vi "Demo Main -translationstage.vi"() -> ()   [LabVIEW 2021]
uses:
  Logo.ctl
  <vilib>/Utility/file.llb/Write Delimited Spreadsheet (string).vi
  <vilib>/Utility/file.llb/Write Delimited Spreadsheet (I64).vi
  <vilib>/Utility/file.llb/Write Delimited Spreadsheet (DBL).vi
  <vilib>/Analysis/NI_AALBase.lvlib
panel:
  in  ".NET Container":refnum<k24>(container)
  in  "MG17Motor":refnum<k7>(container)
  out "ESD":i32=1 caption="Steps\nAdded/Removed"
  in  "ES":i32=1 caption="Add /Remove \nSteps"
  out "Sweep Graph":u32[](graph)
  out "SM":i32 caption="Sweep\nMean"
  out "SN":i32=31 caption="Current Sweep Iteration"
  out "SND":i32=31 caption="Total No. of Sweeps"
  in  "Auto-Sweep":bool
  in  "P8":bool
  out "PC":i32=186 caption="Current \nPosition"
  out "WTD":i32=10000 caption="Wait Time (ms)\nRead Data"
  out "EPD":i32=180 caption="End Position\nRead Data"
  out "SPD":i32 caption="Start Position\nRead Data"
  out "SSD":i32=6 caption="Step Size\nRead Data"
  in  "SP":i32 caption="Start Position (degrees)\n Set Data"
  in  "WT":i32=10000 caption="Wait Time (ms)\n Set Data"
  in  "EP":i32=90 caption="End Position (degrees)\n Set Data"
  in  "P7":bool
  in  "SS":dbl=3.0 caption="Step Size (degrees)\nSet Data"
  in  "Motor Controller\nSerialNumber":string="40837323"
  in  "Export":bool
  out "DB":u32[](array[numeric])=[12, 0, 0, 0, 0, 0, 0, 0, 0, 0, 0, 0, 0, 0, 0, 0]
  out "OVL":bool caption="LED ON : Over Rang Data"
  out "OLD":i32
  out "GN":i32 caption="Gate Number"
  in  "Correction":bool
  in  "Logo":T1
  out "Graph":u32[](graph)=[22]
  in  "Stop":bool
  in  "Start":bool
  in  "P6":bool
  out "RND":i32=10 caption="Read Number\nRead Data"
  in  "P5":bool
  in  "RN":i32=10 caption="Read Number\nSet Data"
  out "PowerD":i32 caption="Power\nRead Data"
  out "ITD":i32=100 caption="Internal Time\nRead Data"
  in  "P4":bool
  in  "P3":bool
  in  "IT":i32=40 caption="Internal Time\nSet Data"
  in  "P2":bool
  out "Handle Number":i32=1331832464
  in  "P1":bool caption="Switch\nPower OFF/Power ON"
  in  "EXIT":bool=TRUE
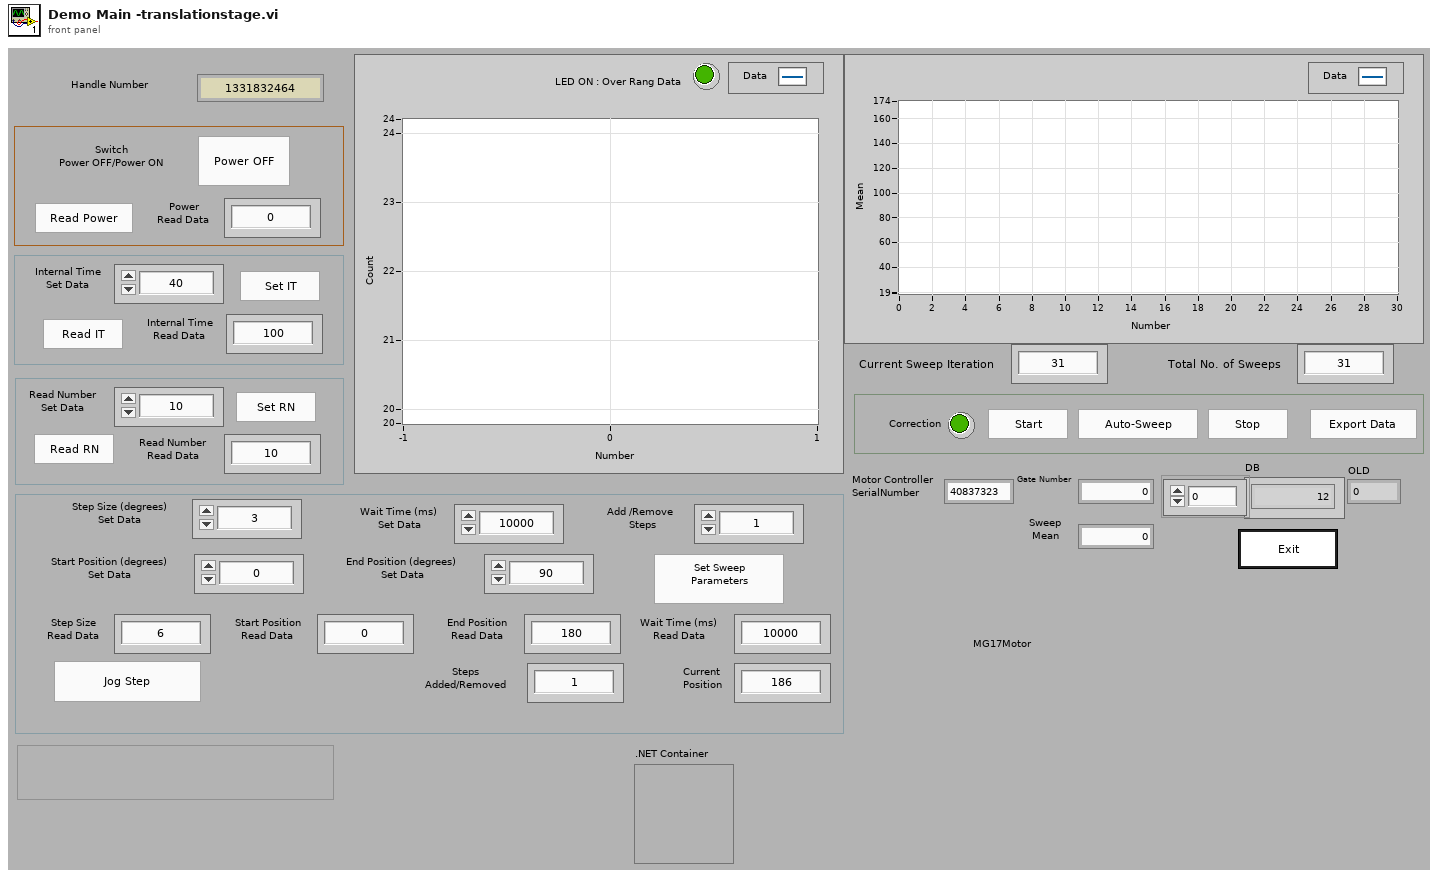
[diagram p1: front panel]
types:
  T1 = typedef "Logo.ctl" = bool
  T2 = enum8{"Enabled", "Disabled", "Disabled and Grayed Out"}
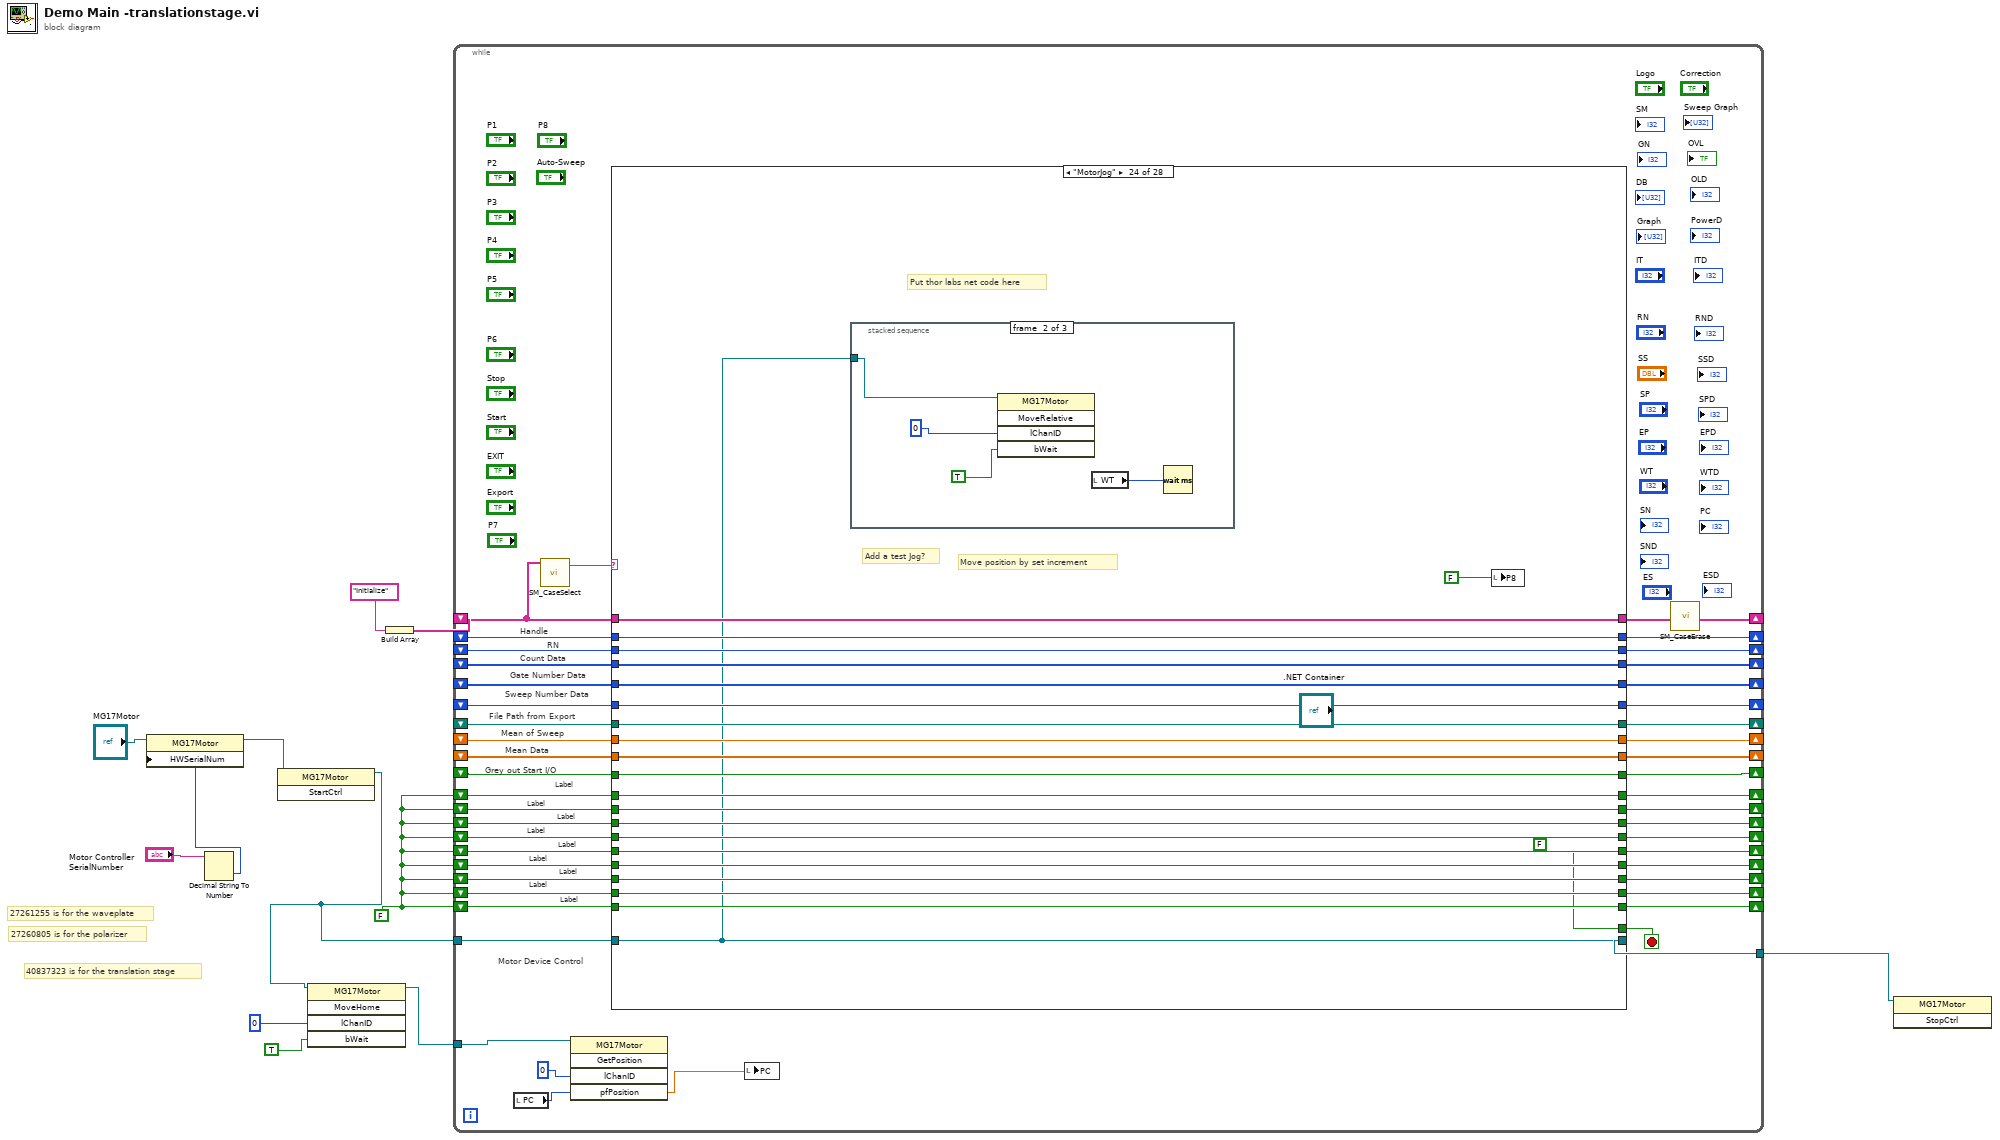
[diagram p0: block diagram]
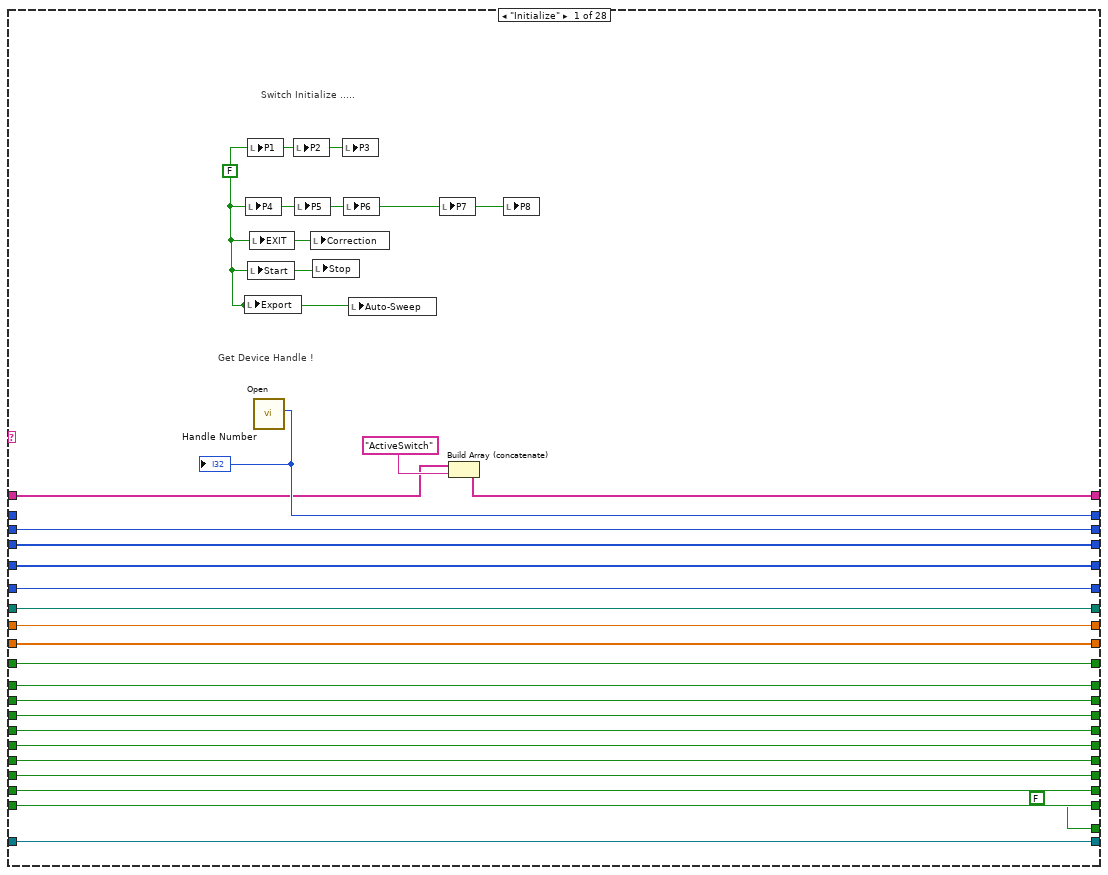
[diagram p2: hidden frame]
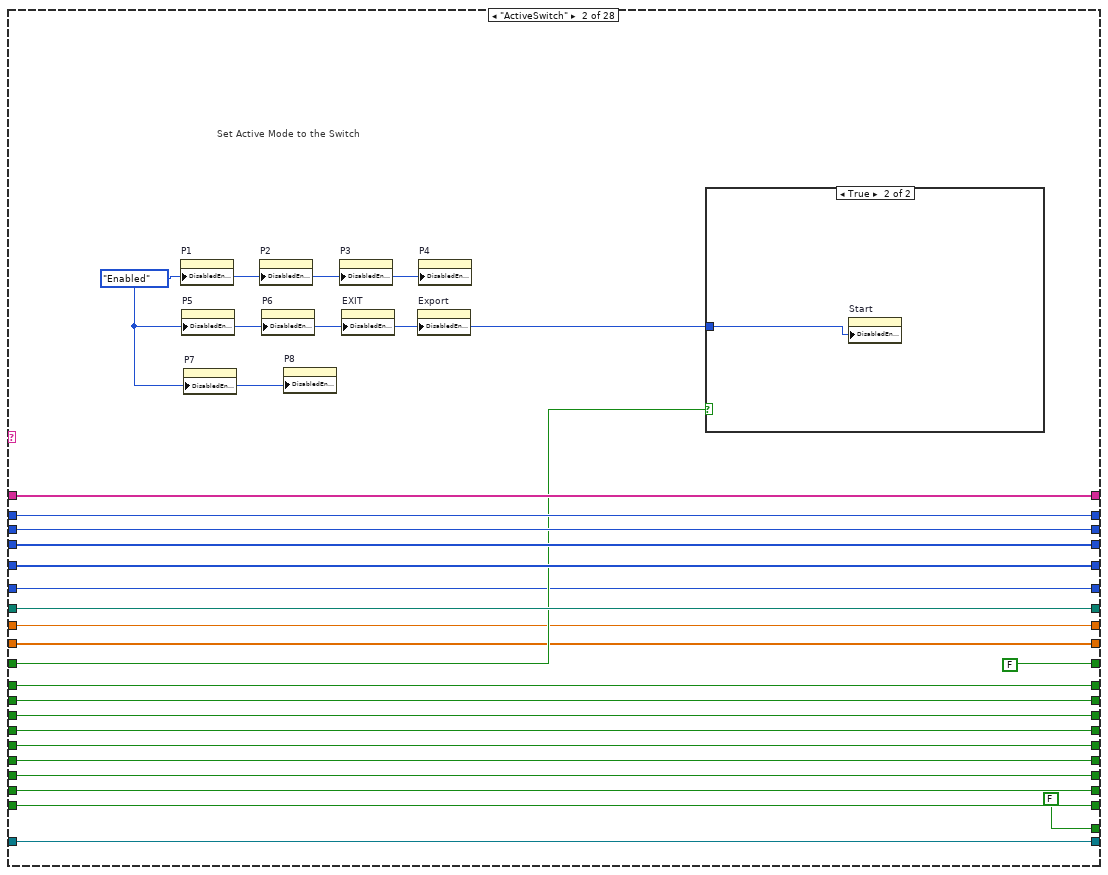
[diagram p3: hidden frame]
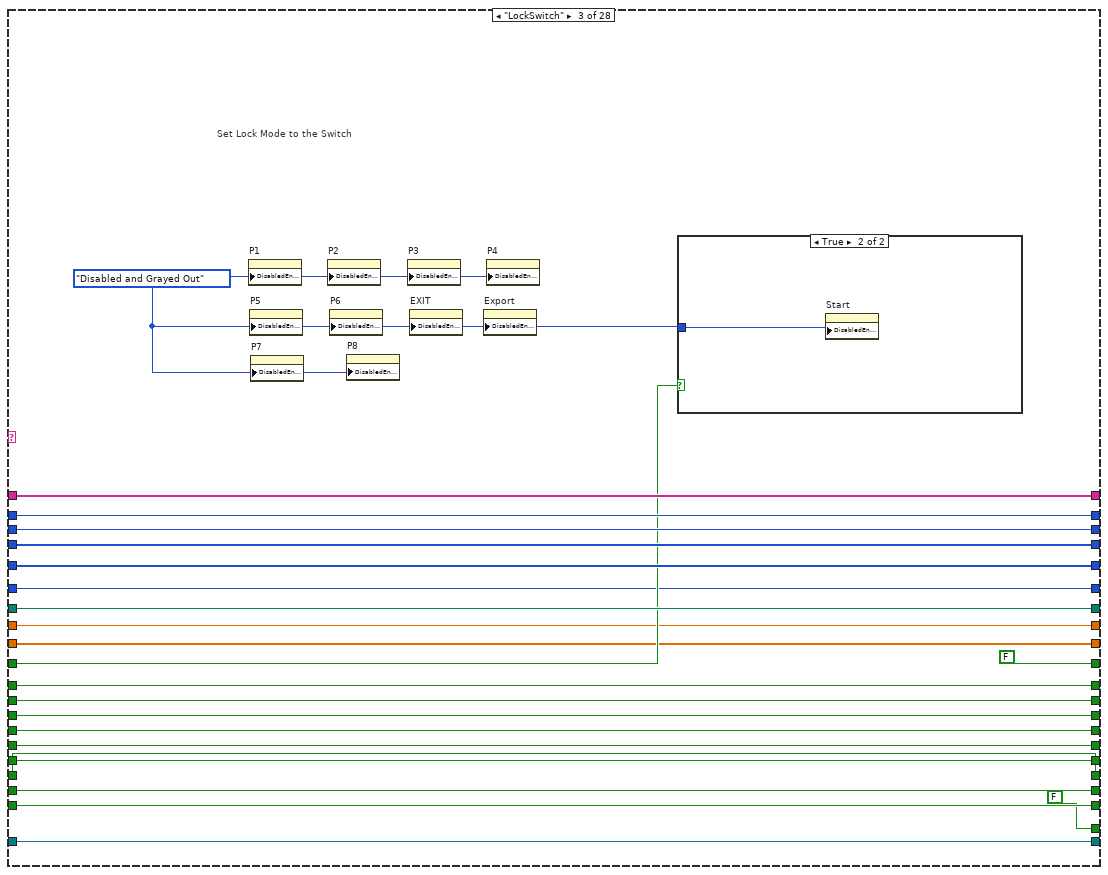
[diagram p5: hidden frame]
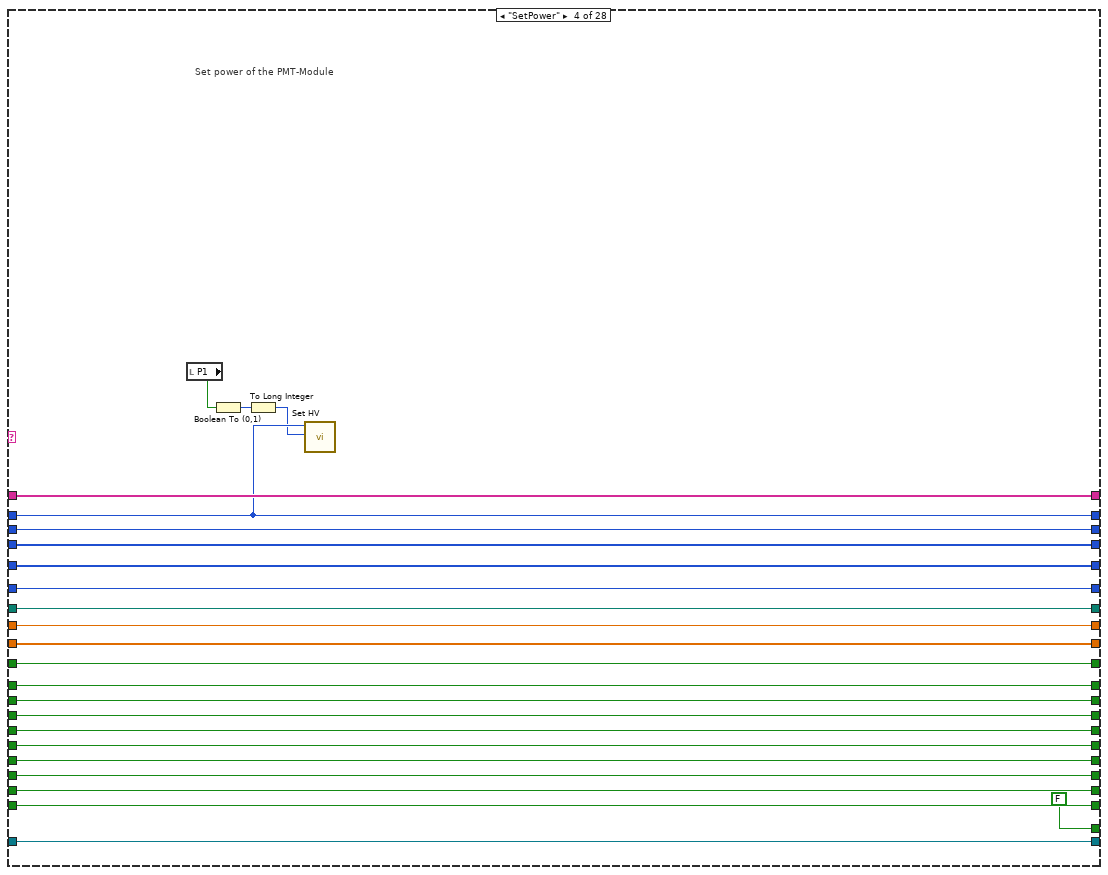
[diagram p7: hidden frame]
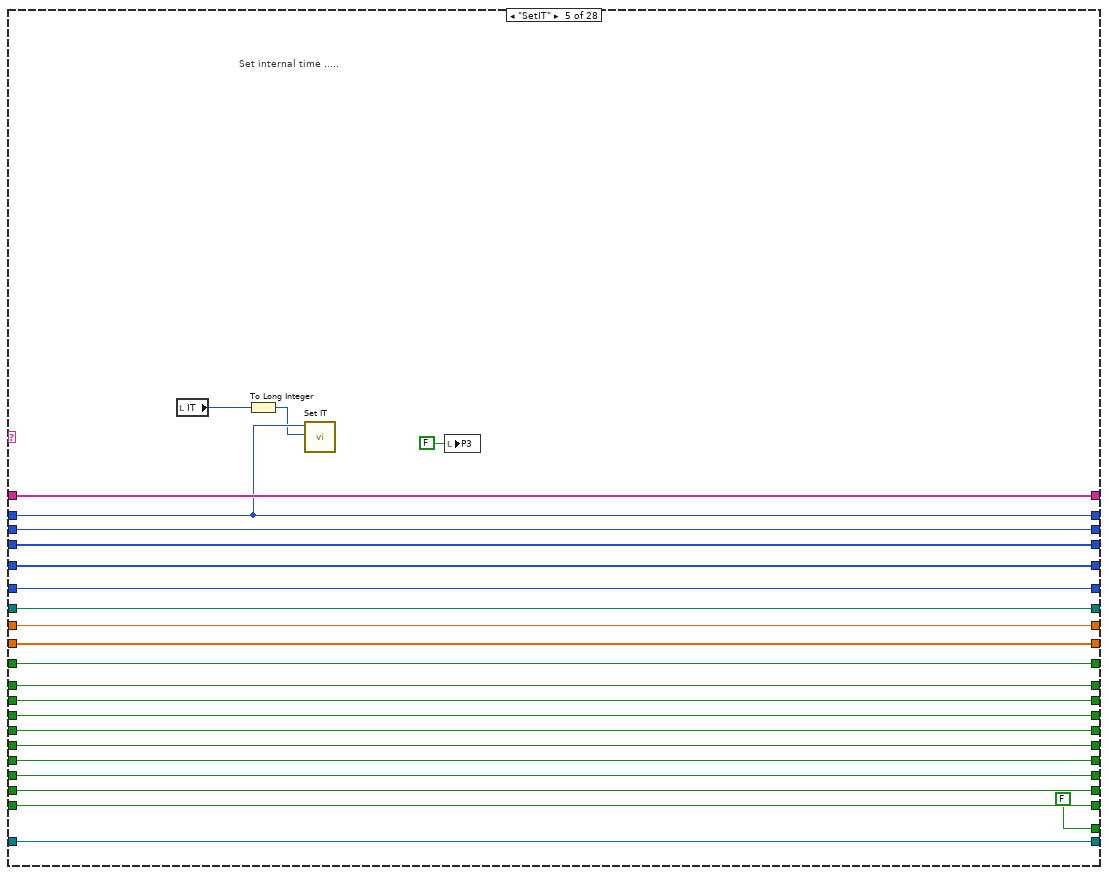
[diagram p8: hidden frame]
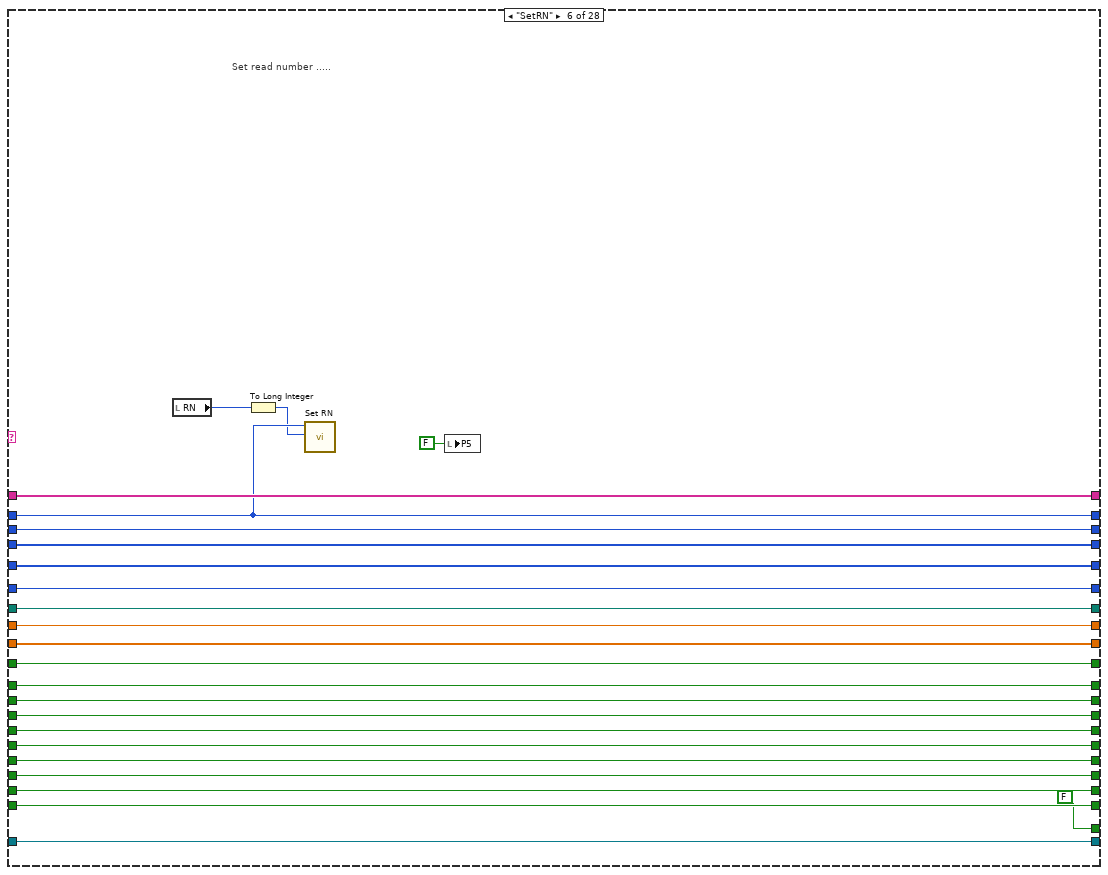
[diagram p9: hidden frame]
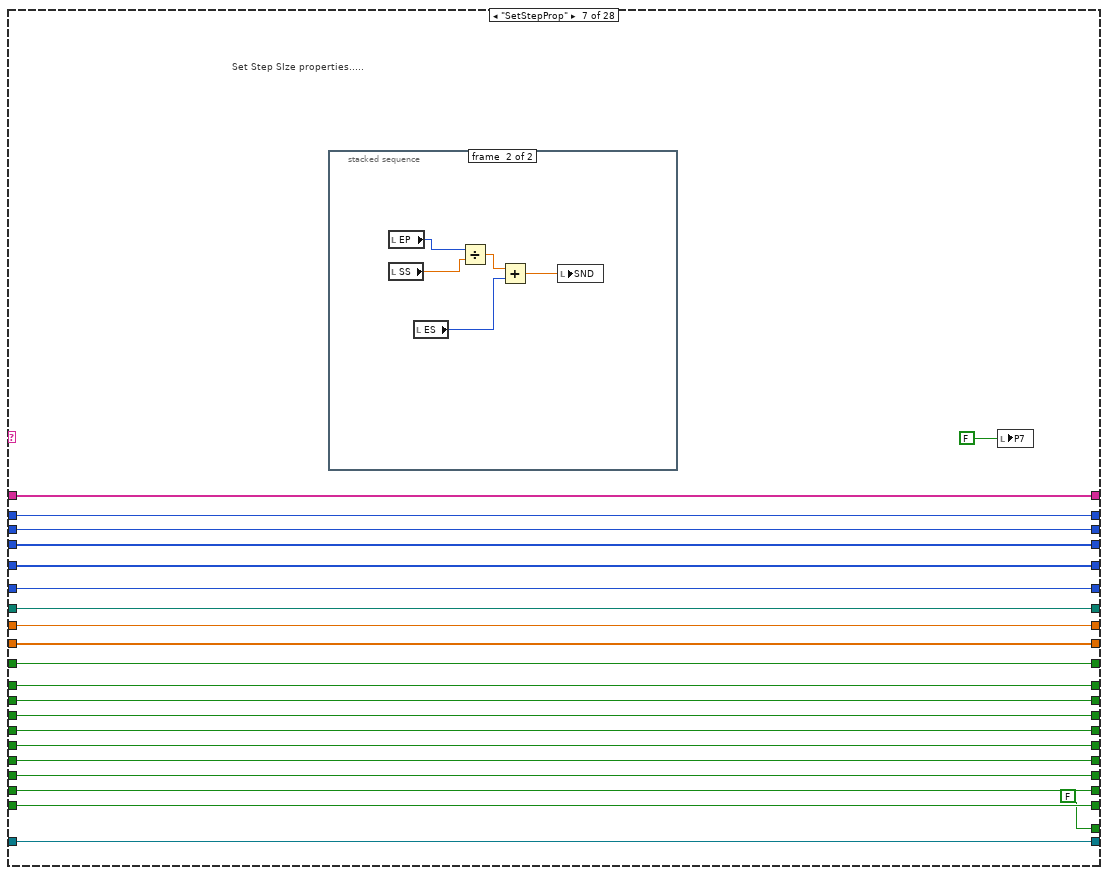
[diagram p10: hidden frame]
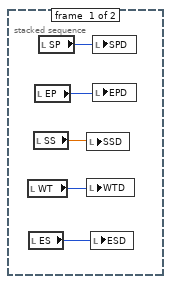
[diagram p11: hidden frame]
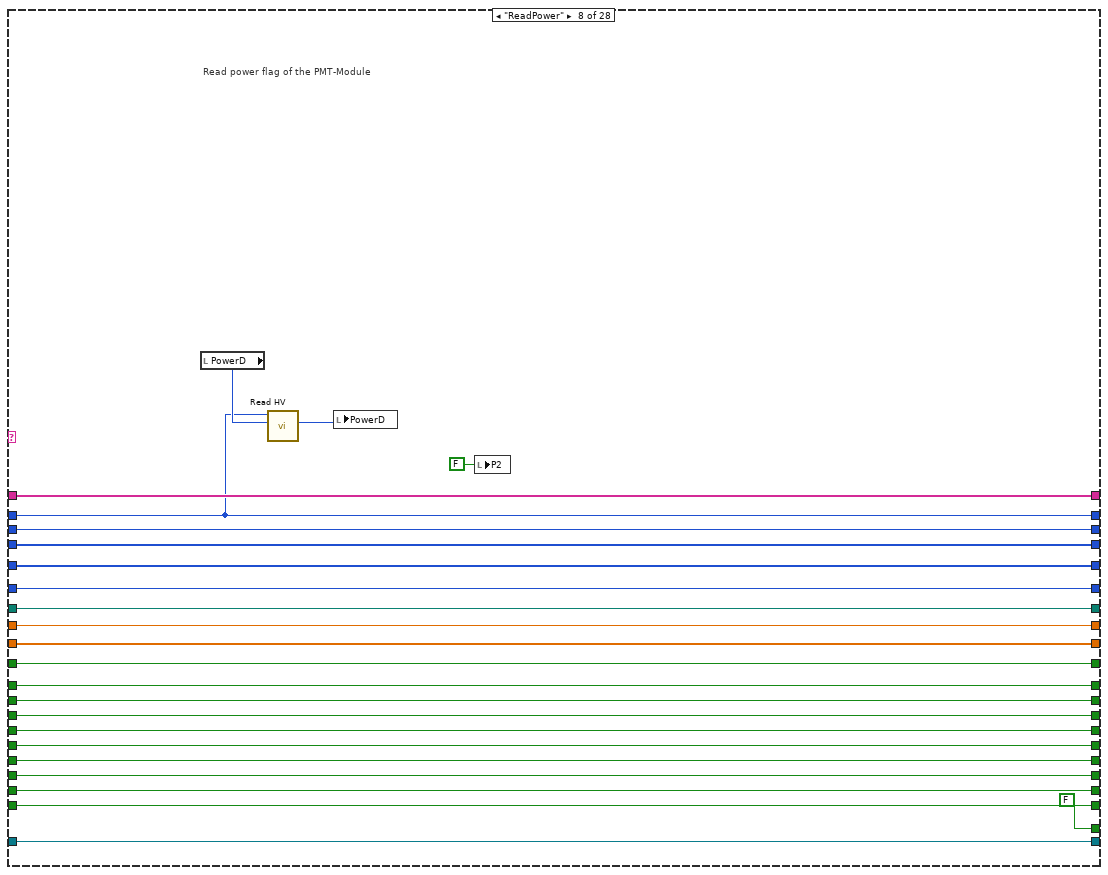
[diagram p12: hidden frame]
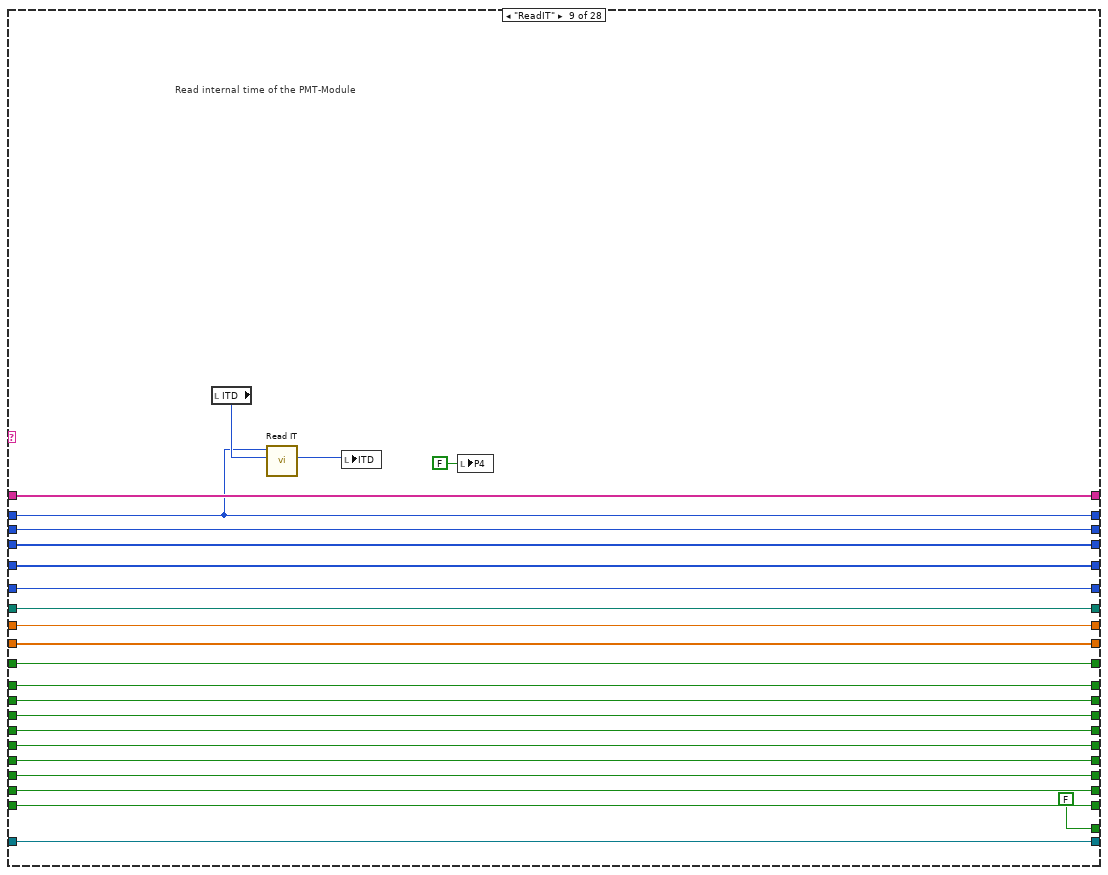
[diagram p13: hidden frame]
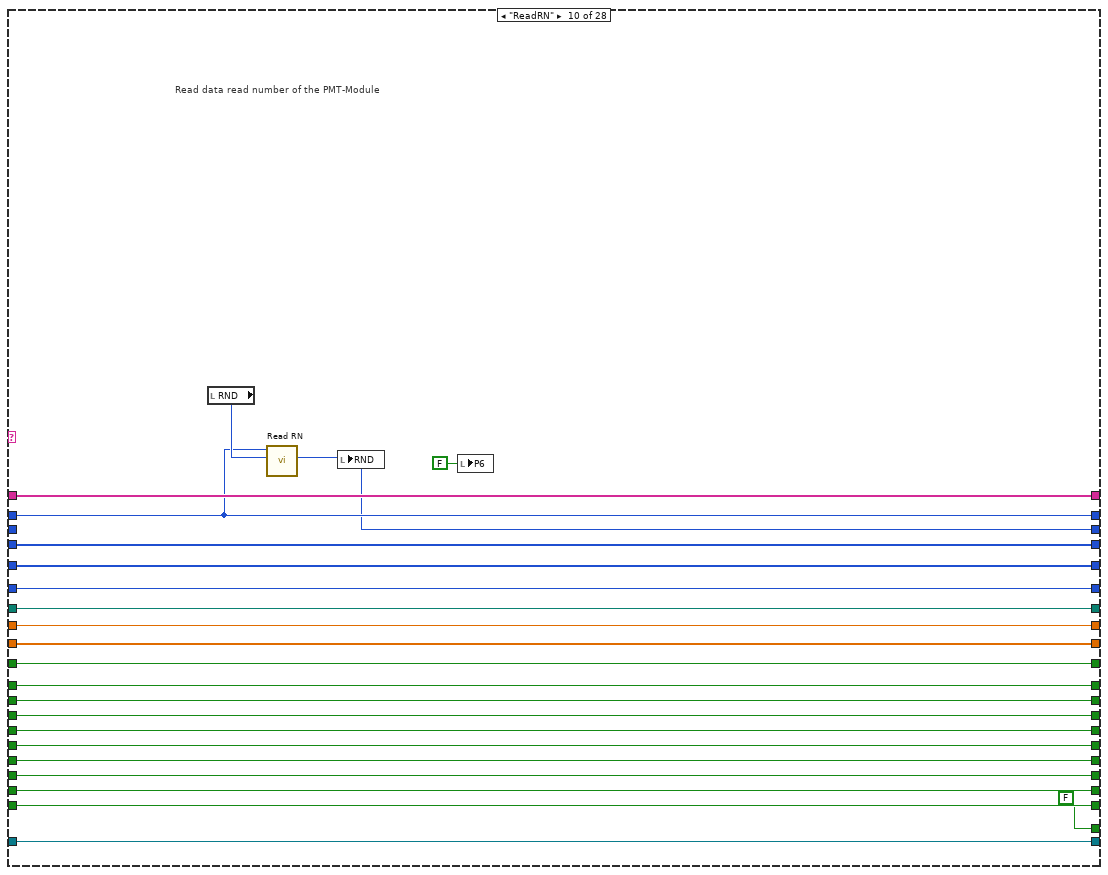
[diagram p14: hidden frame]
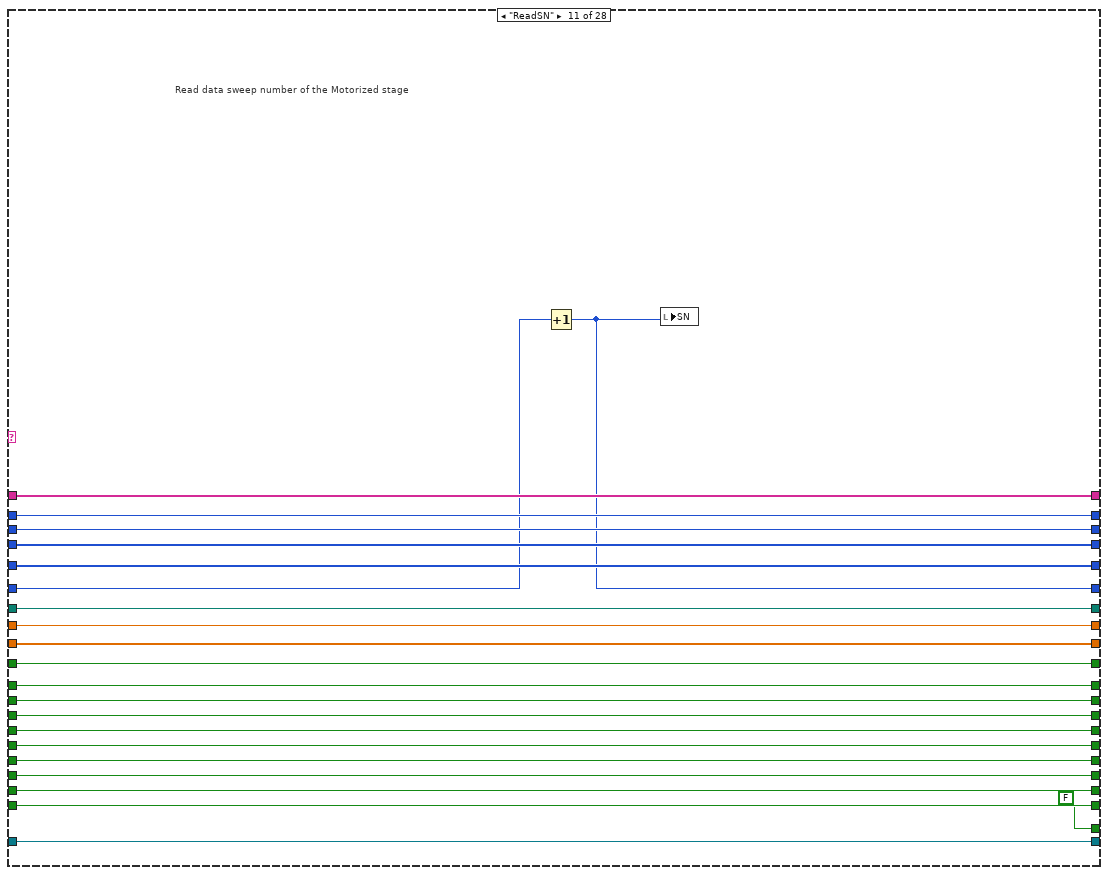
[diagram p15: hidden frame]
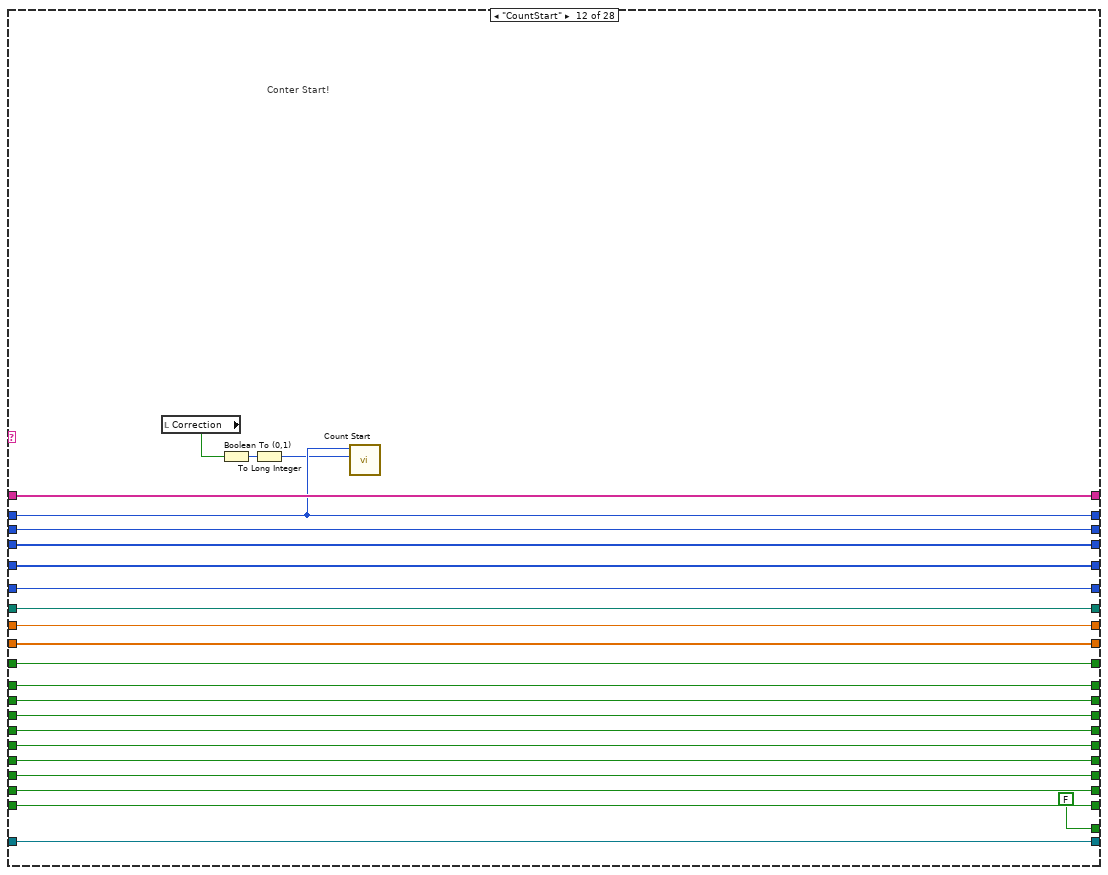
[diagram p16: hidden frame]
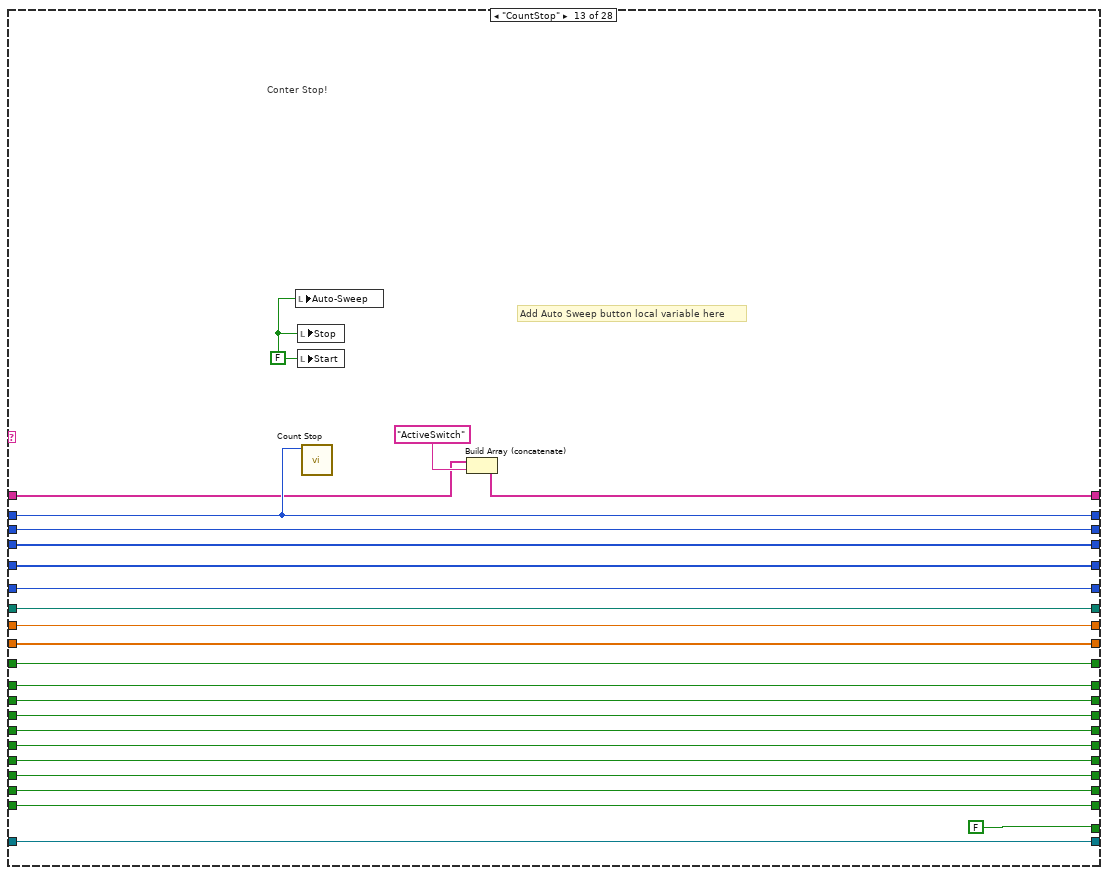
[diagram p17: hidden frame]
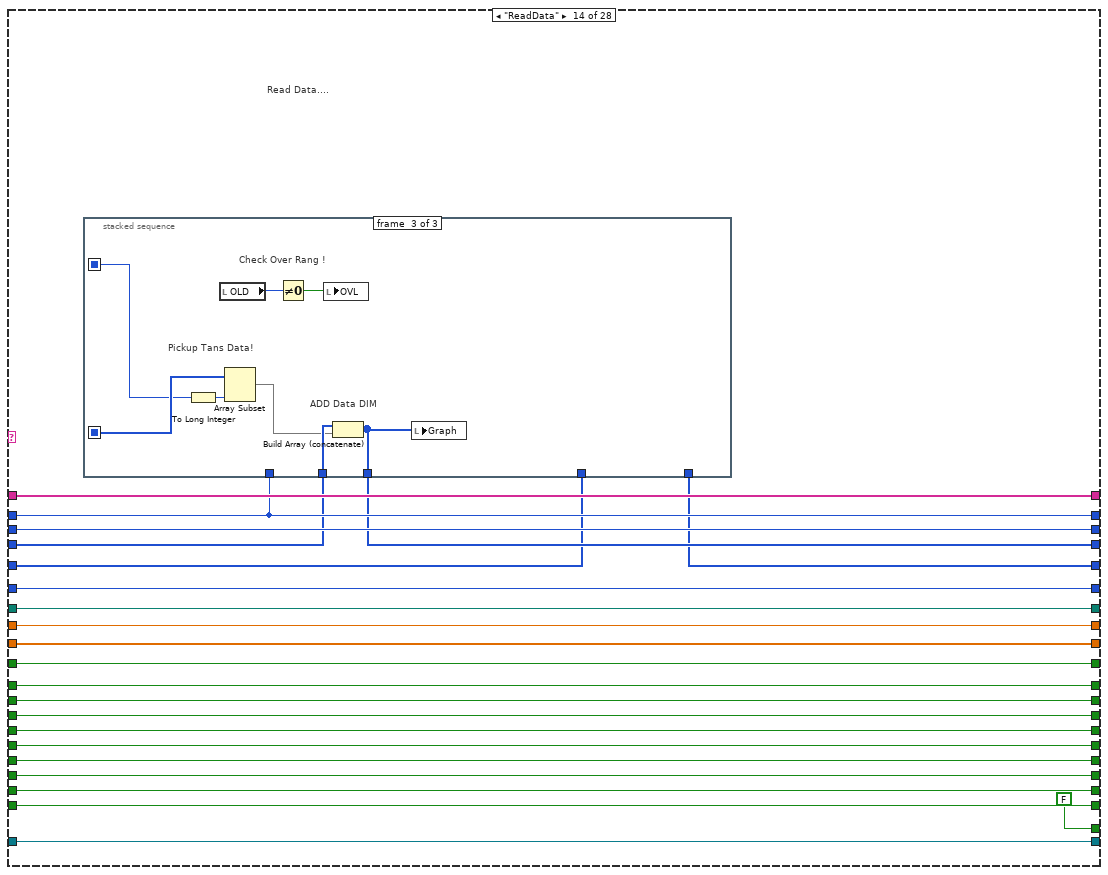
[diagram p18: hidden frame]
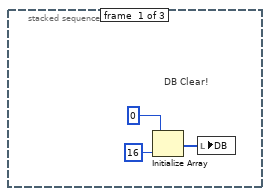
[diagram p19: hidden frame]
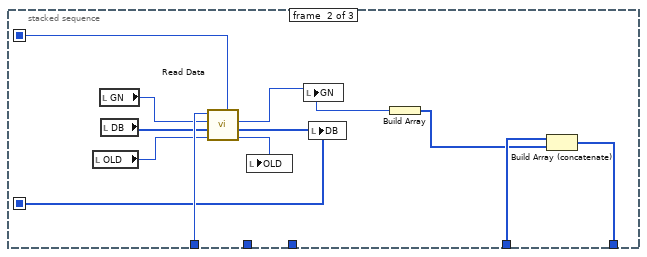
[diagram p20: hidden frame]
diagram:
  w10 = FALSE
  # "40837323 is for the translation stage"
  # "27260805 is for the polarizer"
  # "27261255 is for the waveplate"
  n1 = Decimal String To Number(string="Motor Controller\nSerialNumber") -> (number=w7:i32)  [unwired: 2 in, 1 out]
  n2 = property class="MG17Motor"(reference="MG17Motor", "HWSerialNum"=w7) -> (reference out=w5:refnum<k7>)  [unwired: 1 in, 1 out]
  n3 = invoke class="MG17Motor" method="StartCtrl"(reference=w5) -> (reference out=w4:refnum<k7>)  [unwired: 2 in, 2 out]
  n4 = invoke class="MG17Motor" method="MoveHome"(reference=w4, "lChanID"=0, "bWait"=TRUE) -> (reference out=w3:refnum<k7>)  [unwired: 2 in, 4 out]
  n5 = Build Array("Initialize") -> (w11:string[])
  n6 = while {
    shift-right: [w42] -> _
    shift-left: w10 -> [w43]
    shift-right: [w44] -> _
    shift-left: w10 -> [w45]
    shift-right: [w46] -> _
    shift-left: w10 -> [w47]
    shift-right: [w48] -> _
    shift-left: w10 -> [w49]
    shift-right: [w50] -> _
    shift-left: _ -> [w51]
    shift-right: [w52] -> _
    shift-left: _ -> [w53]
    shift-right: [w54] -> _
    shift-left: _ -> [w55]
    shift-right: [w40] -> _
    shift-left: w10 -> [w41]
    shift-right: [w58] -> _
    shift-left: w10 -> [w59]
    shift-right: [w37] -> _
    shift-left: w11 -> [w56]
    shift-right: [w35] -> _
    shift-left: w10 -> [w36]
    shift-right: [w33] -> _
    shift-left: w10 -> [w34]
    shift-right: [w32] -> _
    shift-left: w10 -> [w31]
    tunnel: w4 -> [w28]
    tunnel: [w27] -> w9
    shift-right: [w30] -> _
    shift-left: _ -> [w29]
    shift-right: [w26] -> _
    shift-left: _ -> [w25]
    shift-right: [w24] -> _
    shift-left: _ -> [w23]
    tunnel: w3 -> [w16]
    shift-right: [w21] -> _
    shift-left: _ -> [w22]
    shift-right: [w20] -> _
    shift-left: _ -> [w19]
    shift-right: [w18] -> _
    shift-left: _ -> [w17]
    stop <- w39 stop-if-true
    # "Mean Data"
    # "Mean of Sweep"
    # "Sweep Number Data"
    # "Grey out Start I/O"
    # "Motor Device Control"
    # "File Path from Export"
    # "Gate Number Data"
    # "Label"
    # "Label"
    # "Label"
    # "Label"
    # "Label"
    # "Label"
    # "Label"
    # "Label"
    # "Label"
    # "Count Data"
    # "RN"
    # "Handle"
    n7 = local read "PC"() -> (w13:i32)
    n8 = call "SM_CaseSelect.vi"("Input"=w56) -> ("Case"=w57:string)  [unwired: 10 out]
    n9 = invoke class="MG17Motor" method="GetPosition"(reference=w16, "lChanID"=0, "pfPosition"=w13) -> ("pfPosition"=w14:sgl)  [unwired: 2 in, 4 out]
    n10 = case shown="\"MotorJog\"" w57 {
      selector: w57 -> [_ _ _ _ _ _ _ _ _ _ _ _ _ _ _ _ _ _ _ _ _ _ _ _ _ _ w937 _]
      tunnel: w59 -> [w83 w106 w130 w155 w179 w203 w225 w259 w283 w306 w328 w352 w376 w399 w443 w474 w500 w540 w578 w647 w700 w751 w781 w802 w835 w884 w955 w976]
      tunnel: [w83 w106 w130 w155 w179 w203 w225 w259 w283 w306 w328 w352 w376 w399 w443 w474 w500 w540 w578 w647 w700 w751 w781 w802 w835 w884 w955 w976] -> w58
      tunnel: w56 -> [w69 w105 w129 w154 w178 w202 w224 w258 w282 w305 w327 w351 w362 w398 w442 w462 w478 w527 w566 w658 w711 w762 w773 w815 w848 w872 w954 w975]
      tunnel: [w68 w105 w129 w154 w178 w202 w224 w258 w282 w305 w327 w351 w361 w398 w442 w461 w477 w528 w567 w658 w711 w762 w772 w815 w848 w869 w954 w975] -> w38
      tunnel: w55 -> [_ w93 w117 w142 w166 w190 w212 w245 w269 w293 w316 w339 w364 w387 w431 w463 w489 w530 w568 w657 w710 w761 w793 w814 w847 w883 w953 w963]
      tunnel: [w71 w93 w117 w142 w166 w190 w212 w245 w269 w293 w316 w339 w364 w387 w431 w463 w489 w530 w568 w657 w710 w761 w793 w814 w847 w883 w953 w963] -> w54
      tunnel: w53 -> [w82 w104 w128 w153 w177 w201 w223 w257 w281 _ w309 w350 w375 w397 w441 w473 w499 w525 w564 w656 w709 w760 w792 w813 w846 w882 w952 w974]
      tunnel: [w82 w104 w128 w153 w177 w201 w223 w257 w281 w291 w309 w350 w375 w397 w441 w473 w499 w525 w564 w656 w709 w760 w792 w813 w846 w882 w952 w974] -> w52
      tunnel: w51 -> [w81 w103 w127 w152 w176 w200 w222 w256 w280 w304 w326 w349 w374 w386 w426 _ _ w521 w562 w632 w685 w736 w791 w812 w845 w868 w951 w973]
      tunnel: [w81 w103 w127 w152 w176 w200 w222 w256 w280 w304 w326 w349 w374 w385 w426 w453 w487 w521 w562 w632 w685 w736 w791 w812 w845 w868 w951 w973] -> w50
      tunnel: w49 -> [w80 w102 w126 w151 w175 w199 w221 w255 w279 w303 w325 w348 w373 w396 w440 w472 w498 w539 w577 w655 w708 w759 w789 w810 w843 w881 w950 w972]
      tunnel: [w80 w102 w126 w151 w175 w199 w221 w255 w279 w303 w325 w348 w373 w396 w440 w472 w498 w539 w577 w655 w708 w759 w789 w810 w843 w881 w950 w972] -> w48
      tunnel: w47 -> [w79 w101 w125 w150 w174 w198 w220 w254 w278 w302 w324 w347 w372 w395 w439 w471 w497 w538 w576 w654 w707 w758 w788 w809 w842 w880 w949 w971]
      tunnel: [w79 w101 w125 w150 w174 w198 w220 w254 w278 w302 w324 w347 w372 w395 w439 w471 w497 w538 w576 w654 w707 w758 w788 w809 w842 w880 w949 w971] -> w46
      tunnel: w45 -> [w78 w100 w124 w149 w173 w197 w219 w253 w277 w301 w323 w346 w371 w394 w438 w470 w496 w537 w575 w653 w706 w757 w787 w808 w841 w879 w948 w970]
      tunnel: [w78 w100 w124 w149 w173 w197 w219 w253 w277 w301 w323 w346 w371 w394 w438 w470 w496 w537 w575 w653 w706 w757 w787 w808 w841 w879 w948 w970] -> w44
      tunnel: w43 -> [w77 w99 w123 w148 w172 w196 w218 w252 w276 w300 w322 w345 w370 w393 w437 w469 w495 w536 w574 w652 w705 w756 w786 w807 w840 w878 w947 w969]
      tunnel: [w77 w99 w123 w148 w172 w196 w218 w252 w276 w300 w322 w345 w370 w393 w437 w469 w495 w536 w574 w652 w705 w756 w786 w807 w840 w878 w947 w969] -> w42
      tunnel: w41 -> [w76 w98 w122 w147 w171 w195 w217 w251 w275 w299 w321 w344 w369 w392 w436 w468 w494 w535 w573 w651 w704 w755 w785 w806 w839 w877 w946 w968]
      tunnel: [w76 w98 w122 w147 w171 w195 w217 w251 w275 w299 w321 w344 w369 w392 w436 w468 w494 w535 w573 w651 w704 w755 w785 w806 w839 w877 w946 w968] -> w40
      tunnel: [FALSE FALSE FALSE FALSE FALSE FALSE FALSE FALSE FALSE FALSE FALSE FALSE FALSE FALSE FALSE FALSE FALSE FALSE FALSE FALSE FALSE FALSE FALSE FALSE FALSE FALSE FALSE TRUE] -> w39
      tunnel: w36 -> [w72 w94 w118 w143 w167 w191 w213 w247 w271 w295 w317 w340 w365 w388 w432 w464 w490 w531 w569 w650 w703 w754 w784 w805 w838 w873 w942 w964]
      tunnel: [w72 w94 w118 w143 w167 w191 w213 w247 w271 w295 w317 w340 w365 w388 w432 w464 w490 w531 w569 w650 w703 w754 w784 w805 w838 w873 w942 w964] -> w35
      tunnel: w34 -> [w74 w96 w120 w145 w169 w193 w215 w249 w273 w297 w319 w342 w367 w390 w434 w466 w492 w533 w571 w649 w702 w753 w783 w804 w837 w875 w944 w966]
      tunnel: [w74 w96 w120 w145 w169 w193 w215 w249 w273 w297 w319 w342 w367 w390 w434 w466 w492 w533 w571 w649 w702 w753 w783 w804 w837 w875 w944 w966] -> w33
      tunnel: [w73 w95 w119 w144 w168 w192 w214 w248 w272 w296 w318 w341 w366 w389 w433 w465 w491 w532 w570 w648 w701 w752 w782 w803 w836 w874 w943 w965] -> w32
      tunnel: w31 -> [w73 w95 w119 w144 w168 w192 w214 w248 w272 w296 w318 w341 w366 w389 w433 w465 w491 w532 w570 w648 w701 w752 w782 w803 w836 w874 w943 w965]
      tunnel: [w67 w92 w116 w138 w162 w186 w211 w242 w266 w290 w315 w335 w360 w384 w425 w453 w487 w520 w561 w627 w680 w731 w790 w811 w844 w867 w936 w962] -> w30
      tunnel: w29 -> [w67 w92 w116 w138 w162 w186 w211 w242 w266 w290 w315 w335 w360 w383 w425 _ _ w520 w561 w627 w680 w731 w790 w811 w844 w867 w936 w962]
      tunnel: w28 -> [w66 w91 w115 w137 w161 w185 w210 w241 w265 w289 w314 w334 w359 w382 w430 w452 w486 w519 w560 w629 w682 w733 w780 w794 w828 w866 w935 w961]
      tunnel: [w66 w91 w115 w137 w161 w185 w210 w241 w265 w289 w314 w334 w359 w382 w430 w452 w486 w519 w560 w629 w682 w733 w780 w794 w828 w866 w935 w961] -> w27
      tunnel: [w65 w90 w114 w136 w160 w184 w208 w240 w264 w288 w313 w333 w358 w381 w429 w451 w485 w518 w559 w620 w676 w727 w769 w800 w833 w865 w934 w960] -> w26
      tunnel: w25 -> [w65 w90 w114 w136 w160 w184 w208 w240 w264 w288 w313 w333 w358 w381 w429 w451 w485 w518 w559 w620 w672 w725 _ w800 w833 w865 w934 w960]
      tunnel: [w64 FALSE FALSE w135 w159 w183 w207 w239 w263 w287 w312 w332 w357 w380 w428 w450 TRUE w517 w558 w622 w675 w726 w778 w799 w832 w864 w933 w959] -> w24
      tunnel: w23 -> [w64 w89 w113 w135 w159 w183 w207 w239 w263 w287 w312 w332 w357 w380 w428 w450 _ w517 _ w622 w675 w726 w778 w799 w832 w864 w933 w959]
      tunnel: w22 -> [w62 w86 w110 w134 w158 w182 w206 w238 w262 w286 w307 w331 w356 w379 w427 w449 w483 w516 w557 w621 w668 w722 _ w795 w831 w863 w932 w958]
      tunnel: [w62 w86 w110 w134 w158 w182 w206 w238 w262 w286 w308 w331 w356 w379 w427 w449 w483 w516 w557 w621 w668 w722 w770 w795 w831 w863 w932 w958] -> w21
      tunnel: [w61 w85 w109 w133 w157 w181 w205 w237 w261 w285 w311 w330 w355 w378 w424 w448 w482 w515 w554 w619 w674 w724 w777 w797 w830 w862 w931 w957] -> w20
      tunnel: w19 -> [w61 w85 w109 w133 w157 w181 w205 w237 w261 w285 w311 w330 w355 w378 w424 w448 w482 w515 w554 w619 _ _ w777 w797 w830 w862 w931 w957]
      tunnel: [w60 w84 w108 w132 w156 w180 w204 w236 w260 w284 w310 w329 w354 w377 w423 w447 w481 w514 w553 w618 w673 w723 w771 w796 w829 w861 w930 w956] -> w18
      tunnel: w17 -> [w60 w84 w108 w132 w156 w180 w204 w236 w260 w284 w310 w329 w354 w377 w422 w447 w481 w514 w553 w618 w673 w723 w771 w796 w829 w861 w930 w956]
      frame "Initialize" {
        w63 = FALSE ("P1")
        # "Get Device Handle !"
        # "Switch Initialize ....."
        n11 = local write "Export"(w63) -> ()
        n12 = local write "P4"(w63) -> ()
        n13 = local write "P1"(w63) -> ()
        n14 = local write "Start"(w63) -> ()
        n15 = local write "EXIT"(w63) -> ()
        n16 = call "Open.vi"() -> ("Handle Number"=w71:i32)  [unwired: 10 in, 1 out]
        "Handle Number" <- w71
        n17 = local write "P2"(w63) -> ()
        n18 = local write "P5"(w63) -> ()
        n19 = local write "Correction"(w63) -> ()
        n20 = local write "Stop"(w63) -> ()
        n21 = local write "P3"(w63) -> ()
        n22 = local write "P6"(w63) -> ()
        n23 = local write "Auto-Sweep"(w63) -> ()
        n24 = local write "P7"(w63) -> ()
        n25 = Build Array (concatenate)(w69, "ActiveSwitch") -> (w68:string[])
        n26 = local write "P8"(w63) -> ()
      }
      frame "ActiveSwitch" {
        w87 = T2."Enabled" ("無効")
        # "Set Active Mode to the Switch"
        n27 = property on="P1" class="Bool (strict)"("DisabledEnum"=w87) -> ()  [unwired: 2 in, 2 out]
        n28 = property on="P5" class="Bool (strict)"("DisabledEnum"=w87) -> ()  [unwired: 2 in, 2 out]
        n29 = property on="P7" class="Bool (strict)"("DisabledEnum"=w87) -> ()  [unwired: 2 in, 2 out]
        n30 = property on="P2" class="Bool (strict)"("DisabledEnum"=w87) -> ()  [unwired: 2 in, 2 out]
        n31 = property on="P6" class="Bool (strict)"("DisabledEnum"=w87) -> ()  [unwired: 2 in, 2 out]
        n32 = property on="P8" class="Bool (strict)"("DisabledEnum"=w87) -> ()  [unwired: 2 in, 2 out]
        n33 = property on="P3" class="Bool (strict)"("DisabledEnum"=w87) -> ()  [unwired: 2 in, 2 out]
        n34 = property on="EXIT" class="Bool (strict)"("DisabledEnum"=w87) -> ()  [unwired: 2 in, 2 out]
        n35 = property on="Export" class="Bool (strict)"("DisabledEnum"=w87) -> ()  [unwired: 2 in, 2 out]
        n36 = property on="P4" class="Bool (strict)"("DisabledEnum"=w87) -> ()  [unwired: 2 in, 2 out]
        n37 = case shown="True" w89 {
          tunnel: w87 -> [_ w107]
          frame False {
          }
          frame True {
            n38 = property on="Start" class="Bool (strict)"("DisabledEnum"=w107) -> ()  [unwired: 2 in, 2 out]
          }
        }
      }
      frame "LockSwitch" {
        w111 = T2."Disabled and Grayed Out" ("無効")
        # "Set Lock Mode to the Switch"
        n39 = property on="P1" class="Bool (strict)"("DisabledEnum"=w111) -> ()  [unwired: 2 in, 2 out]
        n40 = property on="P5" class="Bool (strict)"("DisabledEnum"=w111) -> ()  [unwired: 2 in, 2 out]
        n41 = property on="P7" class="Bool (strict)"("DisabledEnum"=w111) -> ()  [unwired: 2 in, 2 out]
        n42 = property on="P2" class="Bool (strict)"("DisabledEnum"=w111) -> ()  [unwired: 2 in, 2 out]
        n43 = property on="P6" class="Bool (strict)"("DisabledEnum"=w111) -> ()  [unwired: 2 in, 2 out]
        n44 = property on="P8" class="Bool (strict)"("DisabledEnum"=w111) -> ()  [unwired: 2 in, 2 out]
        n45 = property on="P3" class="Bool (strict)"("DisabledEnum"=w111) -> ()  [unwired: 2 in, 2 out]
        n46 = property on="EXIT" class="Bool (strict)"("DisabledEnum"=w111) -> ()  [unwired: 2 in, 2 out]
        n47 = property on="Export" class="Bool (strict)"("DisabledEnum"=w111) -> ()  [unwired: 2 in, 2 out]
        n48 = property on="P4" class="Bool (strict)"("DisabledEnum"=w111) -> ()  [unwired: 2 in, 2 out]
        n49 = case shown="True" w113 {
          tunnel: w111 -> [_ w131]
          frame False {
          }
          frame True {
            n50 = property on="Start" class="Bool (strict)"("DisabledEnum"=w131) -> ()  [unwired: 2 in, 2 out]
          }
        }
      }
      frame "SetPower" {
        # "Set power of the PMT-Module"
        n51 = local read "P1"() -> (w141:bool)
        n52 = Boolean To (0,1)(Boolean=w141) -> (0, 1=w140:i16)
        n53 = To Long Integer(number=w140) -> (32bit integer=w139:i32)
        n54 = call "Set HV.vi"("HV"=w139, "handle"=w142) -> ()  [unwired: 8 in, 2 out]
      }
      frame "SetIT" {
        # "Set internal time ....."
        n55 = local read "IT"() -> (w164:i32)
        n56 = To Long Integer(number=w164) -> (32bit integer=w165:i32)
        n57 = call "Set IT.vi"("IT"=w165, "handle"=w166) -> ()  [unwired: 8 in, 2 out]
        n58 = local write "P3"(FALSE ("P3")) -> ()
      }
      frame "SetRN" {
        # "Set read number ....."
        n59 = local read "RN"() -> (w188:i32)
        n60 = To Long Integer(number=w188) -> (32bit integer=w189:i32)
        n61 = call "Set RN.vi"("RN"=w189, "handle"=w190) -> ()  [unwired: 8 in, 2 out]
        n62 = local write "P5"(FALSE ("P3")) -> ()
      }
      frame "SetStepProp" {
        # "Set Step SIze properties....."
        n63 = stacked-sequence {
          frame #0 {
            n64 = local read "WT"() -> (w227:i32)
            n65 = local read "ES"() -> (w226:i32)
            n66 = local read "SS"() -> (w228:dbl)
            n67 = local read "EP"() -> (w229:i32)
            n68 = local read "SP"() -> (w230:i32)
            n69 = local write "SSD"(w228) -> ()
            n70 = local write "WTD"(w227) -> ()
            n71 = local write "ESD"(w226) -> ()
            n72 = local write "SPD"(w230) -> ()
            n73 = local write "EPD"(w229) -> ()
          }
          frame #1 {
            n74 = local read "EP"() -> (w235:i32)
            n75 = local read "SS"() -> (w234:dbl)
            n76 = local read "ES"() -> (w232:i32)
            n77 = Divide(x=w235, y=w234) -> (x/y=w233:dbl)
            n78 = Add(x=w233, y=w232) -> (x+y=w231:dbl)
            n79 = local write "SND"(w231) -> ()
          }
        }
        n80 = local write "P7"(FALSE) -> ()
      }
      frame "ReadPower" {
        # "Read power flag of the PMT-Module"
        n81 = local read "PowerD"() -> (w246:i32)
        n82 = call "Read HV.vi"("HV"=w246, "handle"=w245) -> ("HV out"=w244:i32)  [unwired: 7 in, 2 out]
        n83 = local write "PowerD"(w244) -> ()
        n84 = local write "P2"(FALSE ("P2")) -> ()
      }
      frame "ReadIT" {
        # "Read internal time of the PMT-Module"
        n85 = local read "ITD"() -> (w270:i32)
        n86 = call "Read IT.vi"("IT"=w270, "handle"=w269) -> ("IT out"=w268:i32)  [unwired: 7 in, 2 out]
        n87 = local write "ITD"(w268) -> ()
        n88 = local write "P4"(FALSE ("P4")) -> ()
      }
      frame "ReadRN" {
        # "Read data read number of the PMT-Module"
        n89 = local read "RND"() -> (w294:i32)
        n90 = call "Read RN.vi"("RN"=w294, "handle"=w293) -> ("RN out"=w291:i32)  [unwired: 7 in, 2 out]
        n91 = local write "RND"(w291) -> ()
        n92 = local write "P6"(FALSE ("P4")) -> ()
      }
      frame "ReadSN" {
        # "Read data sweep number of the Motorized stage"
        n93 = Increment(x=w307) -> (x+1=w308:i32)
        n94 = local write "SN"(w308) -> ()
      }
      frame "CountStart" {
        # "Conter Start!"
        n95 = local read "Correction"() -> (w336:bool)
        n96 = Boolean To (0,1)(Boolean=w336) -> (0, 1=w338:i16)
        n97 = To Long Integer(number=w338) -> (32bit integer=w337:i32)
        n98 = call "Count Start.vi"("Correction"=w337, "handle"=w339) -> ()  [unwired: 8 in, 2 out]
      }
      frame "CountStop" {
        w353 = FALSE ("Start")
        # "Add Auto Sweep button local variable here"
        # "Conter Stop!"
        n99 = local write "Auto-Sweep"(w353) -> ()
        n100 = local write "Stop"(w353) -> ()
        n101 = local write "Start"(w353) -> ()
        n102 = call "Count Stop.vi"("handle"=w364) -> ()  [unwired: 9 in, 2 out]
        n103 = Build Array (concatenate)(w362, "ActiveSwitch") -> (w361:string[])
      }
      frame "ReadData" {
        # "Read Data...."
        n104 = stacked-sequence {
          seq-local: [_ w408 _] -> [_ _ w418]
          seq-local: [_ w407 _] -> [_ _ w419]
          tunnel: w387 -> [_ w413 _]
          tunnel: w386 -> [_ _ w421]
          tunnel: [_ _ w420] -> w385
          tunnel: [_ w403 _] -> w384
          tunnel: w383 -> [_ w406 _]
          frame #0 {
            # "DB Clear!"
            n105 = Initialize Array(u32 0, 16 ("次元サイズ")) -> (w400:u32[])
            n106 = local write "DB"(w400) -> ()
          }
          frame #1 {
            n107 = local read "OLD"() -> (w410:i32)
            n108 = local read "GN"() -> (w412:i32)
            n109 = local read "DB"() -> (w411:u32[])
            n110 = call "Read Data.vi"("OLD"=w410, "DataBuf"=w411, "GateNum"=w412, "handle"=w413) -> ("OLD out"=w409:i32, "DataBuf out"=w407:u32[], "GateNum out"=w405:i32, "function return"=w408:u32)  [unwired: 3 in, 1 out]
            n111 = local write "OLD"(w409) -> ()
            n112 = local write "GN"(w405) -> ()
            n113 = local write "DB"(w407) -> ()
            n114 = Build Array(w405) -> (w404:i32[])
            n115 = Build Array (concatenate)(w406, w404) -> (w403:i32[])
          }
          frame #2 {
            # "Check Over Rang !"
            # "ADD Data DIM"
            # "Pickup Tans Data!"
            n116 = To Long Integer(number=w418) -> (32bit integer=w416:i32)
            n117 = local read "OLD"() -> (w415:i32)
            n118 = Array Subset(array=w419, length=w416) -> (w417:u32[])  [unwired: 1 in]
            n119 = Not Equal To 0?(x=w415) -> (x != 0?=w414:bool)
            n120 = local write "OVL"(w414) -> ()
            n121 = Build Array (concatenate)(w421, w417) -> (w420:u32[])
            n122 = local write "Graph"(w420) -> ()
          }
        }
      }
      frame "AutoReadData" {
        # "add reset for the graph"
        # "Read Data...."
        n123 = stacked-sequence {
          tunnel: w424 -> [w446]
          tunnel: [w445] -> w423
          tunnel: w422 -> [w444]
          frame #0 {
            n124 = Build Array (concatenate)(w444, w446) -> (w445:dbl[])
            n125 = local write "Sweep Graph"(w445) -> ()
          }
        }
      }
      frame "CountInit" {
        w455 = 0
        # "Auto"
        # "Clear Data DIM !"
        n126 = Initialize Array(w455, w455) -> (w453:i32[])
        n127 = Build Array("LockSwitch", "ReadRN", "CountStart", "ReadData", "CheckNumber") -> (w456:string[])
        n128 = Build Array (concatenate)(w462, w456) -> (w461:string[])
      }
      frame "AutoCount|nit!" {
        w488 = 0
        # "Clear Data DIM !"
        n129 = local read "SND"() -> (w475:i32)
        n130 = local read "SN"() -> (w480:i32)
        n131 = Increment(x=w475) -> (x+1=w476:i32)
        n132 = Initialize Array(w488, w488) -> (w487:i32[])
        n133 = Less?(x=w480, y=w476) -> (x < y?=w479:bool)
        n134 = case shown="True" w479 {
          tunnel: w478 -> [w504 w507]
          tunnel: [w502 w506] -> w477
          frame False {
            n135 = Build Array("AutoReadData", "AutoCheckNumber") -> (w503:string[])
            n136 = Build Array (concatenate)(w504, w503) -> (w502:string[])
          }
          frame True {
            n137 = Build Array("LockSwitch", "ReadRN", "CountStart", "ReadData", "AutoCheckNumber") -> (w513:string[])
            n138 = Build Array (concatenate)(w507, w513) -> (w506:string[])
          }
        }
      }
      frame "CheckNumber" {
        # "Add append"
        # "Add Case Strucutre outside\nsimilar to GN,"
        # "Check RN and Data lenbgth,Stop Switch ......"
        n139 = local read "Stop"() -> (w522:bool)
        n140 = local read "GN"() -> (w523:i32)
        n141 = Decrement(x=w525) -> (x-1=w524:i32)
        n142 = Less?(x=w523, y=w524) -> (x < y?=w529:bool)
        n143 = case shown="False" w529 {
          tunnel: [w544 w546] -> w526
          tunnel: w522 -> [_ w545]
          frame False {
            # "\"MotorJog\"; here"
            # "Move \"Active Swith\" to False Condition of Position Number"
            # "Add \"AutoExport Run\" here"
            n144 = local write "Start"(FALSE ("Start")) -> ()
            n145 = Build Array("CountStop", "ActiveSwitch") -> (w544:string[])
          }
          frame True {
            n146 = case shown="False" w545 {
              tunnel: [w548 w550] -> w546
              frame False {
                n147 = Build Array("ReadData", "CheckNumber") -> (w548:string[])
              }
              frame True {
                n148 = Build Array("CountStop") -> (w550:string[])
              }
            }
          }
        }
        n149 = Build Array (concatenate)(w527, w526) -> (w528:string[])
      }
      frame "AutoCheckNumber" {
        # "Add append"
        # "Add Case Strucutre outside\nsimilar to GN,"
        # "Check RN and Data lenbgth,Stop Switch ......"
        n150 = local read "Stop"() -> (w563:bool)
        n151 = local read "SND"() -> (w552:i32)
        n152 = local read "SN"() -> (w556:i32)
        n153 = Less?(x=w556, y=w552) -> (x < y?=w555:bool)
        n154 = case shown="False" w555 {
          tunnel: [w580 w590] -> w565
          tunnel: w564 -> [_ w589]
          tunnel: w563 -> [_ w586]
          tunnel: [TRUE w585] -> w558
          frame False {
            w584 = FALSE ("Start")
            n155 = local write "Auto-Sweep"(w584) -> ()
            n156 = local write "Start"(w584) -> ()
            n157 = Build Array("CountStop", "AutoExportSweep", "ActiveSwitch") -> (w580:string[])
          }
          frame True {
            n158 = local read "GN"() -> (w587:i32)
            n159 = Decrement(x=w589) -> (x-1=w588:i32)
            n160 = Less?(x=w587, y=w588) -> (x < y?=w591:bool)
            n161 = case shown="False" w591 {
              tunnel: [w593 w609] -> w590
              tunnel: w586 -> [w594 w608]
              tunnel: [w592 w607] -> w585
              frame False {
                # "\"MotorJog\"; here"
                # "Move \"Active Swith\" to False Condition of Position Number"
                # "Add \"AutoExport Run\" here"
                n162 = case shown="False" w594 {
                  tunnel: [w600 w605] -> w593
                  tunnel: [FALSE TRUE] -> w592
                  frame False {
                    n163 = Build Array("CountStop", "AutoExportRun", "AutoReadData", "ReadSN", "MotorJog", "AutoCount|nit!") -> (w600:string[])
                  }
                  frame True {
                    n164 = local write "Auto-Sweep"(TRUE) -> ()
                    n165 = Build Array("CountStop") -> (w605:string[])
                  }
                }
              }
              frame True {
                n166 = case shown="False" w608 {
                  tunnel: [w612 w616] -> w609
                  tunnel: [FALSE TRUE] -> w607
                  frame False {
                    n167 = Build Array("ReadData", "AutoCheckNumber") -> (w612:string[])
                  }
                  frame True {
                    n168 = Build Array("CountStop") -> (w616:string[])
                    n169 = local write "Auto-Sweep"(TRUE) -> ()
                  }
                }
              }
            }
          }
        }
        n170 = Build Array (concatenate)(w566, w565) -> (w567:string[])
      }
      frame "Export" {
        # "For Auto Export also add mean waveform"
        # "Get mean Data into 1D array Shift register for waveform"
        # "Gate Number is just number of count measurements"
        # "time...using array size"
        # "time...using array size"
        n171 = Array Size(array=w632) -> (size(s)=w644:i32)
        n172 = for {
          N: w644 -> [_]
          tunnel: [w659] -> w631 mode=indexing
          i -> [w661]
          n173 = local read "ITD"() -> (w663:i32)
          n174 = Add(x=1, y=w661) -> (x+y=w662:i32)
          n175 = Multiply(x=w663, y=w662) -> (x*y=w659:i32)
        }
        n176 = call <vilib>:"Std Deviation and Variance.vi"("X"=w632) -> ("mean"=w625:dbl, "standard deviation"=w624:dbl)  [unwired: 1 in, 1 out]
        n177 = Build Array(w625, w624) -> (w623:dbl[])
        n178 = Build Array(w627, w631, w632) -> (w642:u32[][])
        n179 = call-poly <vilib>:"Write Delimited Spreadsheet.vi"("1D data"=string[] ["Gate  No.", "Time [ms]", "Counts"], "append to file? (new file:F)"=FALSE, "transpose? (no:F)"=FALSE) -> ("new file path (Not A Path if cancelled)"=w641:path)  [unwired: 11 in, 1 out]
        n180 = call-poly <vilib>:"Write Delimited Spreadsheet.vi"("file path (dialog if empty)"=w641, "2D data"=w642, "append to file? (new file:F)"=TRUE, "transpose? (no:F)"=TRUE) -> ("new file path (Not A Path if cancelled)"=w637:path)  [unwired: 10 in, 1 out]
        n181 = call-poly <vilib>:"Write Delimited Spreadsheet.vi"("file path (dialog if empty)"=w637, "1D data"=string[] ["Mean", "Std. Dev."], "append to file? (new file:F)"=TRUE, "transpose? (no:F)"=FALSE) -> ("new file path (Not A Path if cancelled)"=w633:path)  [unwired: 10 in, 1 out]
        n182 = call-poly <vilib>:"Write Delimited Spreadsheet.vi"("file path (dialog if empty)"=w633, "1D data"=w623, "append to file? (new file:F)"=TRUE, "transpose? (no:F)"=FALSE) -> ()  [unwired: 10 in, 2 out]
        n183 = local write "Export"(FALSE) -> ()
      }
      frame "AutoExportRun" {
        # "For Auto Export also add mean waveform"
        # "Get mean Data into 1D array Shift register for waveform"
        # "Gate Number is just number of count measurements"
        # "time...using array size"
        # "time...using array size"
        n184 = Array Size(array=w685) -> (size(s)=w697:i32)
        n185 = for {
          N: w697 -> [_]
          tunnel: [w717] -> w684 mode=indexing
          i -> [w719]
          n186 = local read "ITD"() -> (w721:i32)
          n187 = Add(x=1, y=w719) -> (x+y=w720:i32)
          n188 = Multiply(x=w721, y=w720) -> (x*y=w717:i32)
        }
        n189 = flat-sequence {
          tunnel: w668 -> [w716]
          tunnel: [w712] -> w667
          frame #0 {
            n190 = local read "SS"() -> (w715:dbl)
            n191 = Multiply(x=w716, y=w715) -> (x*y=w713:dbl)
            n192 = local read "SP"() -> (w714:i32)
            n193 = Add(x=w714, y=w713) -> (x+y=w712:dbl)
          }
        }
        n194 = call <vilib>:"Std Deviation and Variance.vi"("X"=w685) -> ("mean"=w674:dbl, "standard deviation"=w678:dbl)  [unwired: 1 in, 1 out]
        n195 = Build Array(w674, w678) -> (w677:dbl[])
        n196 = Number To Decimal String(number=w667) -> (decimal integer string=w666:string)  [unwired: 1 in]
        n197 = Build Array(w680, w684, w685) -> (w695:u32[][])
        n198 = Build Array (concatenate)(string[] ["Angle (deg)"], w666) -> (w664:string[])
        n199 = call-poly <vilib>:"Write Delimited Spreadsheet.vi"("file path (dialog if empty)"=w672, "1D data"=w664, "append to file? (new file:F)"=TRUE, "transpose? (no:F)"=FALSE) -> ("new file path (Not A Path if cancelled)"=w671:path)  [unwired: 10 in, 1 out]
        n200 = call-poly <vilib>:"Write Delimited Spreadsheet.vi"("file path (dialog if empty)"=w671, "1D data"=string[] ["Gate  No.", "Time [ms]", "Counts"], "append to file? (new file:F)"=TRUE, "transpose? (no:F)"=FALSE) -> ("new file path (Not A Path if cancelled)"=w694:path)  [unwired: 10 in, 1 out]
        n201 = call-poly <vilib>:"Write Delimited Spreadsheet.vi"("file path (dialog if empty)"=w694, "2D data"=w695, "append to file? (new file:F)"=TRUE, "transpose? (no:F)"=TRUE) -> ("new file path (Not A Path if cancelled)"=w690:path)  [unwired: 10 in, 1 out]
        n202 = call-poly <vilib>:"Write Delimited Spreadsheet.vi"("file path (dialog if empty)"=w690, "1D data"=string[] ["Mean", "Std. Dev."], "append to file? (new file:F)"=TRUE, "transpose? (no:F)"=FALSE) -> ("new file path (Not A Path if cancelled)"=w686:path)  [unwired: 10 in, 1 out]
        n203 = call-poly <vilib>:"Write Delimited Spreadsheet.vi"("file path (dialog if empty)"=w686, "1D data"=w677, "append to file? (new file:F)"=TRUE, "transpose? (no:F)"=FALSE) -> ("new file path (Not A Path if cancelled)"=w676:path)  [unwired: 10 in, 1 out]
        n204 = local write "Export"(FALSE) -> ()
      }
      frame "AutoExportSweep" {
        # "For Auto Export also add mean waveform"
        # "Get mean Data into 1D array Shift register for waveform"
        # "Gate Number is just number of count measurements"
        # "time...using array size"
        # "time...using array size"
        n205 = Array Size(array=w723) -> (size(s)=w748:i32)
        n206 = for {
          N: w748 -> [_]
          tunnel: [w766] -> w735 mode=indexing
          i -> [w763]
          n207 = local read "SS"() -> (w767:dbl)
          n208 = Multiply(x=w767, y=w763) -> (x*y=w764:dbl)
          n209 = local read "SP"() -> (w765:i32)
          n210 = Add(x=w765, y=w764) -> (x+y=w766:dbl)
        }
        n211 = call <vilib>:"Std Deviation and Variance.vi"("X"=w723) -> ("mean"=w724:dbl, "standard deviation"=w729:dbl)  [unwired: 1 in, 1 out]
        n212 = Build Array(w724, w729) -> (w728:dbl[])
        n213 = Build Array(w735, w723) -> (w746:dbl[][])
        n214 = call-poly <vilib>:"Write Delimited Spreadsheet.vi"("file path (dialog if empty)"=w725, "1D data"=string[] ["Angle Itr.", "Counts Mean", ""], "append to file? (new file:F)"=TRUE, "transpose? (no:F)"=FALSE) -> ("new file path (Not A Path if cancelled)"=w745:path)  [unwired: 10 in, 1 out]
        n215 = call-poly <vilib>:"Write Delimited Spreadsheet.vi"("file path (dialog if empty)"=w745, "2D data"=w746, "append to file? (new file:F)"=TRUE, "transpose? (no:F)"=TRUE) -> ("new file path (Not A Path if cancelled)"=w741:path)  [unwired: 10 in, 1 out]
        n216 = call-poly <vilib>:"Write Delimited Spreadsheet.vi"("file path (dialog if empty)"=w741, "1D data"=string[] ["Mean", "Std. Dev."], "append to file? (new file:F)"=TRUE, "transpose? (no:F)"=FALSE) -> ("new file path (Not A Path if cancelled)"=w737:path)  [unwired: 10 in, 1 out]
        n217 = call-poly <vilib>:"Write Delimited Spreadsheet.vi"("file path (dialog if empty)"=w737, "1D data"=w728, "append to file? (new file:F)"=TRUE, "transpose? (no:F)"=FALSE) -> ("new file path (Not A Path if cancelled)"=w727:path)  [unwired: 10 in, 1 out]
        n218 = local write "Export"(FALSE) -> ()
      }
      frame "AutoSweep" {
        w770 = 0
        # "1. Create a file path (Send two strings, \"SetPosition\" and \"AutoCount|nit!\")\n2. Send to \"SetPosition\"\n2.1. Will create a Position Number Shift register\n2.2. Move stage to initial position, allow time to complete movement or add delay\n3. Send to \"AutoCount|nit!\"\n3.1. \"AutoCount|nit!\" is clone of \"Count|nit!\" but sends to \"AutoCheckNumber\", not \"CheckNumber\n3.1.1. \"AutoCheckNumber\" will check if end position, or run condition is met then send \"CountStop\" and \"ActiveSwitch\"\n3.1.2. \"AutoCheck Number\" will allow \"CountStop\" to be sent via Stop Boolean\n3.1.3. \"AutoCheckNumber\" will upon END of one run will run \"AutoExportRun\" to set file path\n3.1.3.1. \"AutoExportRun\" will add a data point to Mean Waveform after Count Stop\n3.1.4. \"AutoCheckNumber\" will upon END of sweep will run \"AutoExportSweep\" then issue \"ActiveSwitch\"\n3.1.4.1. \"AutoExportSweep\" will append final Mean Sweep waveform to file path before \"CountStop\";\"ActiveSwitch\"\n4. If End condition not met; \"MotorJog\"; \"AutoCount|nit!\"....repeats\n4.1. Will move to next position by set increment, with .net code, add delay to allow it to arrive at position"
        # "Create a File path here\nSend switch case string \"SetPosition\", which has a position number switch register"
        # "1.Position Set, create a file path\n2. Count|nit!---duplicate and create auto counter, add read sweep data for auto read\n2.0.1Checknumber end, change active switch to Auto export\n3. Auto Export ... need to make \n3.0.2Auto Export end, send to read sweep data (mean, stdev for per sweep)\n3.Export\n4.check end position, check end condition met\n5.met>end;not end >continue\n6. Jog motor\n7.repeat from 2."
        # "Create Motor Controls for setting Homing, Step size for angle, idle time(if required),"
        n219 = local write "SN"(w770) -> ()
        n220 = call-poly <vilib>:"Write Delimited Spreadsheet.vi"("append to file? (new file:F)"=FALSE) -> ("new file path (Not A Path if cancelled)"=w769:path)  [unwired: 13 in, 1 out]
        n221 = Build Array("SetPosition", "AutoCount|nit!") -> (w775:string[])
        n222 = Build Array (concatenate)(w773, w775) -> (w772:string[])
      }
      frame "MotorJog" {
        # "Move position by set increment"
        # "Add a test Jog?"
        # "Put thor labs net code here"
        n223 = stacked-sequence {
          tunnel: w794 -> [w818 w820 w826]
          frame #0 {
            n224 = local read "SSD"() -> (w817:i32)
            n225 = invoke class="MG17Motor" method="SetRelMoveDist"(reference=w818, "lChanID"=0, "fRelDist"=w817) -> ()  [unwired: 2 in, 5 out]
          }
          frame #1 {
            n226 = invoke class="MG17Motor" method="MoveRelative"(reference=w820, "lChanID"=0, "bWait"=TRUE) -> ()  [unwired: 2 in, 5 out]
            n227 = local read "WT"() -> (w821:i32)
            n228 = Wait (ms)(milliseconds to wait=w821) -> ()  [unwired: 1 out]
          }
          frame #2 {
            n229 = local read "PC"() -> (w823:i32)
            n230 = invoke class="MG17Motor" method="GetPosition"(reference=w826, "lChanID"=0, "pfPosition"=w823) -> ("pfPosition"=w824:sgl)  [unwired: 2 in, 4 out]
            n231 = Wait (ms)(milliseconds to wait=50) -> ()  [unwired: 1 out]
            n232 = local write "PC"(w824) -> ()
          }
        }
        n233 = local write "P8"(FALSE) -> ()
      }
      frame "SetPosition" {
        n234 = stacked-sequence {
          tunnel: w828 -> [w850 w853 w859]
          frame #0 {
            n235 = local read "SPD"() -> (w849:i32)
            n236 = invoke class="MG17Motor" method="SetAbsMovePos"(reference=w850, "lChanID"=0, "fAbsPos"=w849) -> ()  [unwired: 2 in, 5 out]
          }
          frame #1 {
            n237 = invoke class="MG17Motor" method="MoveAbsolute"(reference=w853, "lChanID"=0, "bWait"=TRUE) -> ()  [unwired: 2 in, 5 out]
            n238 = local read "WT"() -> (w855:i32)
            n239 = Wait (ms)(milliseconds to wait=w855) -> ()  [unwired: 1 out]
          }
          frame #2 {
            n240 = local read "PC"() -> (w856:i32)
            n241 = invoke class="MG17Motor" method="GetPosition"(reference=w859, "lChanID"=0, "pfPosition"=w856) -> ("pfPosition"=w857:sgl)  [unwired: 2 in, 4 out]
            n242 = local write "PC"(w857) -> ()
            n243 = Wait (ms)(milliseconds to wait=50) -> ()  [unwired: 1 out]
          }
        }
      }
      frame "", "Idle" {
        n244 = event shown="[8] \"Start\": Value Change" {
          selector: _ -> [_ _ _ _ _ _ _ _ _ _ _ _ _]
          dyn-events: _ -> [_ _ _ _ _ _ _ _ _ _ _ _ _]
          timeout: _ -> [_ _ _ _ _ _ _ _ _ _ _ _ _]
          tunnel: w872 -> [w887 w890 w893 w897 w901 w905 w909 w913 w916 w918 w921 w924 w927]
          tunnel: [w885 w889 w892 w896 w900 w904 w908 w912 w915 w917 w920 w923 w928] -> w870
          event Menu Selection (User) {
            n245 = event-data() -> ("ItemTag"=w886:string)  [unwired: 1 out]
            n246 = Build Array (concatenate)(w887, w886) -> (w885:string[])
          }
          event "EXIT": Value Change {
            n247 = event-data() -> ()  [unwired: 7 out]
            n248 = Build Array (concatenate)(w890, "Exit") -> (w889:string[])
          }
          event "P1": Value Change {
            n249 = event-data() -> ()  [unwired: 7 out]
            n250 = Build Array (concatenate)(w893, "SetPower") -> (w892:string[])
          }
          event "P2": Value Change {
            n251 = event-data() -> ()  [unwired: 7 out]
            n252 = Build Array (concatenate)(w897, "ReadPower") -> (w896:string[])
            n253 = Wait (ms)(milliseconds to wait=u32 200 ("ミリ秒待機時間")) -> ()  [unwired: 1 out]
          }
          event "P3": Value Change {
            n254 = event-data() -> ()  [unwired: 7 out]
            n255 = Build Array (concatenate)(w901, "SetIT") -> (w900:string[])
            n256 = Wait (ms)(milliseconds to wait=u32 200 ("ミリ秒待機時間")) -> ()  [unwired: 1 out]
          }
          event "P4": Value Change {
            n257 = event-data() -> ()  [unwired: 7 out]
            n258 = Build Array (concatenate)(w905, "ReadIT") -> (w904:string[])
            n259 = Wait (ms)(milliseconds to wait=u32 200 ("ミリ秒待機時間")) -> ()  [unwired: 1 out]
          }
          event "P5": Value Change {
            n260 = event-data() -> ()  [unwired: 7 out]
            n261 = Build Array (concatenate)(w909, "SetRN") -> (w908:string[])
            n262 = Wait (ms)(milliseconds to wait=u32 200 ("ミリ秒待機時間")) -> ()  [unwired: 1 out]
          }
          event "P6": Value Change {
            n263 = event-data() -> ()  [unwired: 7 out]
            n264 = Build Array (concatenate)(w913, "ReadRN") -> (w912:string[])
            n265 = Wait (ms)(milliseconds to wait=u32 200 ("ミリ秒待機時間")) -> ()  [unwired: 1 out]
          }
          event "Start": Value Change {
            n266 = event-data() -> ()  [unwired: 7 out]
            n267 = Build Array (concatenate)(w916, "CountInit") -> (w915:string[])
          }
          event "Export": Value Change {
            n268 = event-data() -> ()  [unwired: 7 out]
            n269 = Build Array (concatenate)(w918, "Export") -> (w917:string[])
          }
          event "P7": Value Change {
            n270 = event-data() -> ()  [unwired: 7 out]
            n271 = Build Array (concatenate)(w921, "SetStepProp") -> (w920:string[])
          }
          event "P8": Value Change {
            n272 = event-data() -> ()  [unwired: 7 out]
            n273 = Build Array (concatenate)(w924, "MotorJog") -> (w923:string[])
          }
          event "Auto-Sweep": Value Change {
            n274 = event-data() -> ()  [unwired: 7 out]
            n275 = Build Array (concatenate)(w927, "AutoSweep") -> (w928:string[])
            n276 = Wait (ms)(milliseconds to wait=200) -> ()  [unwired: 1 out]
          }
        }
        n277 = Build Array (concatenate)("", w870) -> (w869:string[])
      }
      frame "Error", Default {
        n278 = Concatenate Strings("Error  Case Name .....", "\r\n", w937) -> (w939:string)
        n279 = One Button Dialog(message=w939) -> (true=w938:bool)  [unwired: 1 out]
        n280 = stacked-sequence {
          tunnel: w938 -> [_]
          frame #0 {
            n281 = Stop() -> ()  [unwired: 1 out]
          }
        }
      }
      frame "Exit" {
        # "See you again ......"
        n282 = call "Close.vi"("Handle"=w963) -> ()  [unwired: 9 in, 2 out]
      }
    }
    n283 = local write "PC"(w14) -> ()
    n284 = call "SM_CaseErase.vi"("Input"=w38) -> ("Output"=w37:string[])  [unwired: 10 out]
  }
  n285 = invoke class="MG17Motor" method="StopCtrl"(reference=w9) -> ()  [unwired: 2 in, 3 out]
